vi "create.vi"(8 "error in (no error)":errorcluster, 11 "Create":dbl) -> (0 "error out":errorcluster, 3 "UserEditableAmount out":refnum<class "UserEditableAmount.lvclass">)   [LabVIEW 2020, in "UserEditableAmount.lvclass"]
uses:
  UserEditableAmount.lvclass
  UserEditableAmount.lvclass/UserEditableAmount.ctl
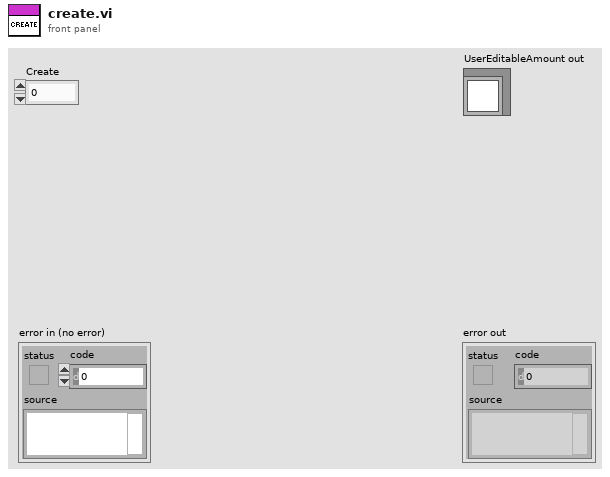
[diagram p1: front panel]
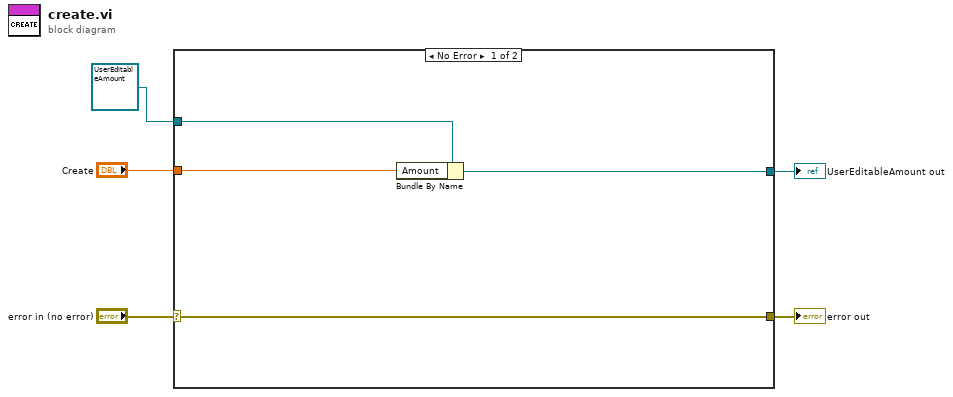
[diagram p0: block diagram]
diagram:
  n1 = case shown="No Error" "error in (no error)" {
    selector: "error in (no error)" -> [w9 w11]
    tunnel: [w9 w11] -> w4
    tunnel: [w7 w10] -> w3
    tunnel: "Create" -> [w8 _]
    tunnel: refnum<class "UserEditableAmount.lvclass"> refnum ("UserEditableAmount") -> [w6 w10]
    frame No Error {
      n2 = Bundle By Name(cluster=w6, "Amount"=w8) -> (w7:refnum<class "UserEditableAmount.lvclass">)
    }
    frame Error {
    }
  }
  "error out" <- w4
  "UserEditableAmount out" <- w3
